vi "servo set pulse.vi"(8 "error in":errorcluster, 10 "servo pulse(us)":dbl, 11 "Enum":T1) -> (0 "error out":errorcluster)   [LabVIEW 2019, in "my FPGA lib.lvlib"]
uses:
  my FPGA lib.lvlib
  Servo.enum.ctl
  <vilib>/Utility/error.llb/Error Cluster From Error Code.vi
  <vilib>/rvi/errors/niLvFpgaAdjustHostInterfaceError.vi
  <vilib>/ErrorRing/Error Ring.xnode
  <vilib>/rvi/interface/nirviReadWriteControl/nirviReadWriteControl.xnode
  FPGA/FPPGA.ctl
  NiFpgaLv.dll
  <vilib>/rvi/interface/Simulation/niFpgaSimulationCallBeginRW.vi
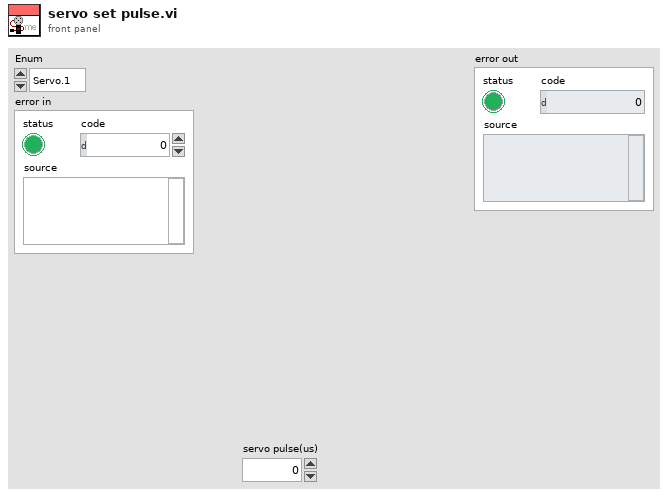
[diagram p1: front panel]
types:
  T1 = typedef "my FPGA lib.lvlib/Servo.enum.ctl" = enum16{"Servo.1", "Servo.2", "Servo.3", "Servo.4"}
  T2 = typedef "my FPGA lib.lvlib/FPPGA.ctl" = refnum<k20>
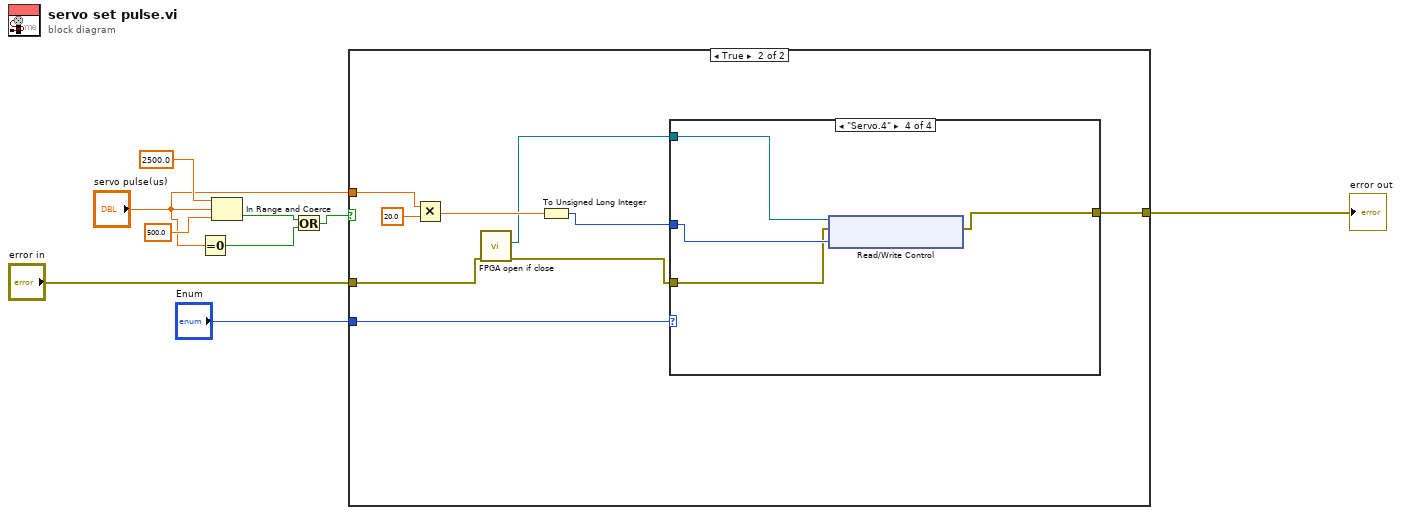
[diagram p0: block diagram]
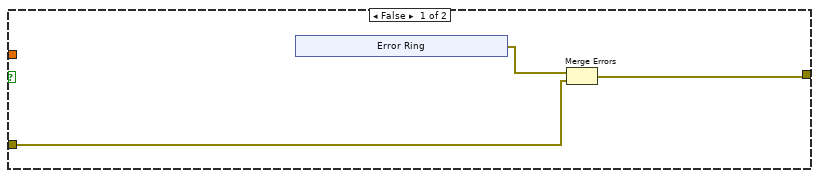
[diagram p2: hidden frame]
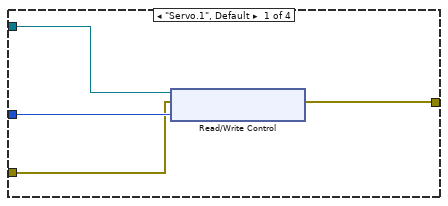
[diagram p3: hidden frame]
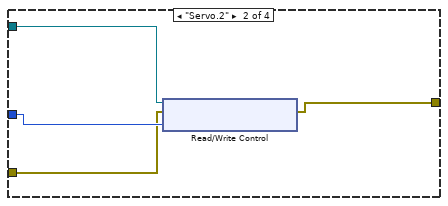
[diagram p4: hidden frame]
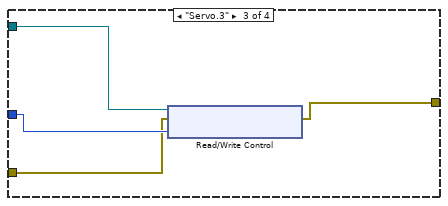
[diagram p5: hidden frame]
diagram:
  n1 = Equal To 0?(x="servo pulse(us)") -> (x = 0?=w2:bool)
  n2 = In Range and Coerce(upper limit=2500.0, x="servo pulse(us)", lower limit=500.0) -> (In Range?=w3:bool)  [unwired: 1 out]
  n3 = Or(x=w3, y=w2) -> (x .or. y?=w1:bool)
  n4 = case shown="True" w1 {
    tunnel: "servo pulse(us)" -> [_ w25]
    tunnel: "Enum" -> [_ w24]
    tunnel: "error in" -> [w10 w19]
    tunnel: [w12 w21] -> w5
    frame False {
      n5 = xnode "Error Ring"() -> ("error out"=w11:errorcluster)
      n6 = Merge Errors(w11, w10) -> (w12:errorcluster)
    }
    frame True {
      n7 = Multiply(x=w25, y=20.0) -> (x*y=w23:dbl)
      n8 = call "FPGA open if close.vi"("error in"=w19) -> ("error out"=w20:errorcluster, "FPGA VI Reference Out"=w18:T2)  [unwired: 9 in]
      n9 = To Unsigned Long Integer(number=w23) -> (unsigned 32bit integer=w22:u32)
      n10 = case shown="\"Servo.4\"" w24 {
        tunnel: w18 -> [w30 w34 w38 w42]
        tunnel: w22 -> [w29 w33 w37 w41]
        tunnel: w20 -> [w28 w32 w36 w40]
        tunnel: [w27 w31 w35 w39] -> w21
        frame "Servo.1", Default {
          n11 = xnode "Read/Write Control"("FPGA VI Reference In"=w30, "error in"=w28, "Servo1.pulse(0.05us)"=w29) -> ("error out"=w27:errorcluster)  [unwired: 1 out]
        }
        frame "Servo.2" {
          n12 = xnode "Read/Write Control"("FPGA VI Reference In"=w34, "error in"=w32, "Servo2.pulse(0.05us)"=w33) -> ("error out"=w31:errorcluster)  [unwired: 1 out]
        }
        frame "Servo.3" {
          n13 = xnode "Read/Write Control"("FPGA VI Reference In"=w38, "error in"=w36, "Servo3.pulse(0.05us)"=w37) -> ("error out"=w35:errorcluster)  [unwired: 1 out]
        }
        frame "Servo.4" {
          n14 = xnode "Read/Write Control"("FPGA VI Reference In"=w42, "error in"=w40, "Servo4.pulse(0.05us)"=w41) -> ("error out"=w39:errorcluster)  [unwired: 1 out]
        }
      }
    }
  }
  "error out" <- w5
